vi "修改地址.vi"() -> ()   [LabVIEW 2015]
uses:
  <vilib>/Instr/_visa.llb/VISA Configure Serial Port (Instr).vi
panel:
  out "Baudrate":i32
  out "COM":string
  in  "MyIndex":u8
  in  "当前地址":string="\u0000"
  out "OK?":bool
  out "Send":string
  out "Read":string
  in  "目标地址":string="\u0002"
  out "error out":errorcluster caption="错误输出"
  in  "error in (no error)":errorcluster caption="错误输入（无错误）"
  # "注：当前485只有一个LED分析仪的时候使用，当前地址填写为00时，可直接设置地址；\n若有多个LED分析仪需要分开设置，或者输入当前地址一个个进行设置。地址设置成功后需要断电重启LED分析仪。"
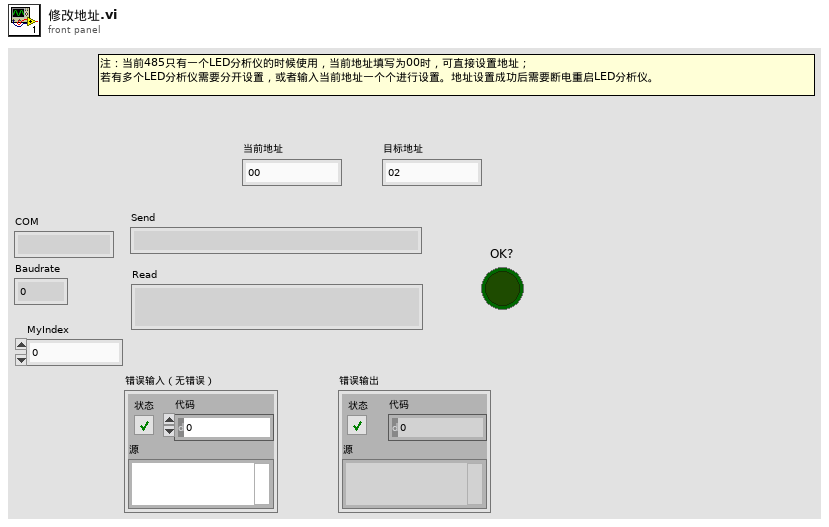
[diagram p1: front panel]
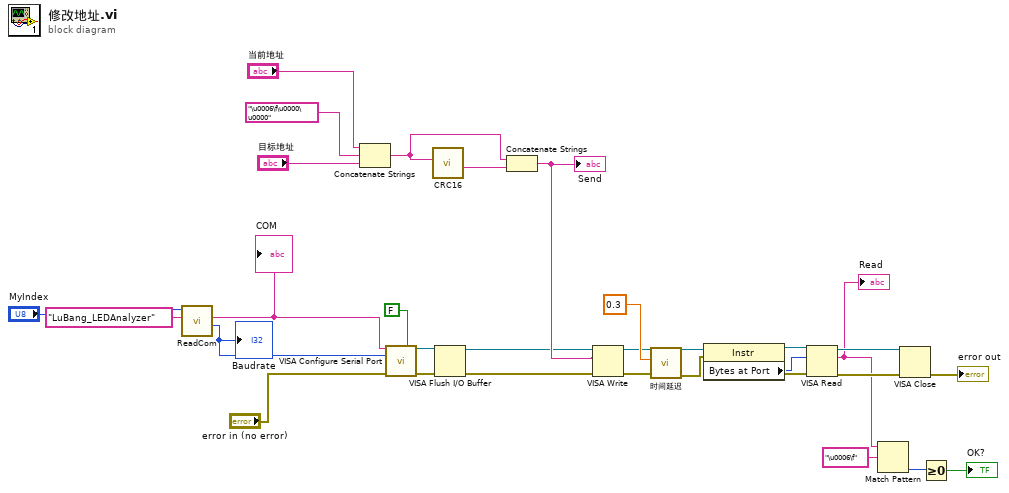
[diagram p0: block diagram]
diagram:
  n1 = call "ReadCom.vi"("仪器名称"="LuBang_LEDAnalyzer", "MyIndex"="MyIndex") -> ("Baudrate"=w1:i32, "COM"=w2:string)  [unwired: 7 in, 1 out]
  "COM" <- w2
  "Baudrate" <- w1
  n2 = Concatenate Strings("当前地址", "\u0006\f\u0000\u0000", "目标地址") -> (w24:string)
  n3 = call-poly "VISA Configure Serial Port"("VISA resource name"=w2, "Enable Termination\nChar (T)"=FALSE ("Enable Termination\nChar (T)"), "baud rate (9600)"=w1, "error in (no error)"="error in (no error)") -> ("VISA resource name out"=w27:refnum<visa-resource-name>, "error out"=w28:errorcluster)  [unwired: 10 in]
  n4 = call "CRC16.vi"("输入字符串"=w24) -> ("CRC16(String)"=w23:string)  [unwired: 9 in, 1 out]
  n5 = VISA Flush I/O Buffer(VISA resource name=w27, error in (no error)=w28) -> (VISA resource name out=w21:refnum<visa-resource-name>, error out=w20:errorcluster)  [unwired: 1 in]
  n6 = Concatenate Strings(w24, w23) -> (w22:string)
  "Send" <- w22
  n7 = VISA Write(VISA resource name=w21, write buffer=w22, error in (no error)=w20) -> (VISA resource name out=w16:refnum<visa-resource-name>, error out=w19:errorcluster)  [unwired: 1 out]
  n8 = call "时间延迟"("error in (no error)"=w19, "Delay Time (s)"=0.3) -> ("error out"=w5:errorcluster)  [unwired: 9 in]
  n9 = property class="Instr"(reference=w16, error in=w5) -> (reference out=w15:refnum<visa-resource-name>, error out=w17:errorcluster, "Bytes at Port"=w14:u32)
  n10 = VISA Read(VISA resource name=w15, byte count=w14, error in (no error)=w17) -> (VISA resource name out=w12:refnum<visa-resource-name>, read buffer=w10:string, error out=w13:errorcluster)  [unwired: 1 out]
  "Read" <- w10
  n11 = Match Pattern(string=w10, regular expression="\u0006\f" ("正则表达式")) -> (offset past match=w8:i32)  [unwired: 1 in, 3 out]
  n12 = VISA Close(VISA resource name=w12, error in (no error)=w13) -> (error out=→"error out":errorcluster)
  n13 = Greater Or Equal To 0?(x=w8) -> (x >= 0?=→"OK?":bool)
